vi "NFC Mngr.vi"(7 "Mngr Action":T1, 8 "error in (no error)":errorcluster, 10 "Python Version":string, 11 "Reader SN":string="21121521200223") -> (0 "error out":errorcluster, 3 "Cartridge SN":string, 4 "Connected":bool)   [LabVIEW 2018]
uses:
  NFC Mngr.ctl
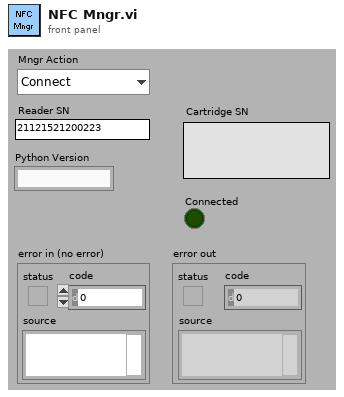
[diagram p1: front panel]
types:
  T1 = typedef "NFC Mngr.ctl" = enum16{"Connect", "Read SN", "Close"}
  T2 = enum16{"Init", "Reset", "Read", "Update", "Close"}
  T3 = cluster{"negative limit switch":bool, "positive limit switch":bool, "home switch":bool, "position marker":bool, "device enable":bool, "quick stop":bool, "general purpose J":bool, "general purpose I":bool, "general purpose H":bool, "general purpose G":bool, "general purpose F":bool, "general purpose E":bool, "general purpose D":bool, "general purpose C":bool, "general purpose B":bool, "general purpose A":bool}
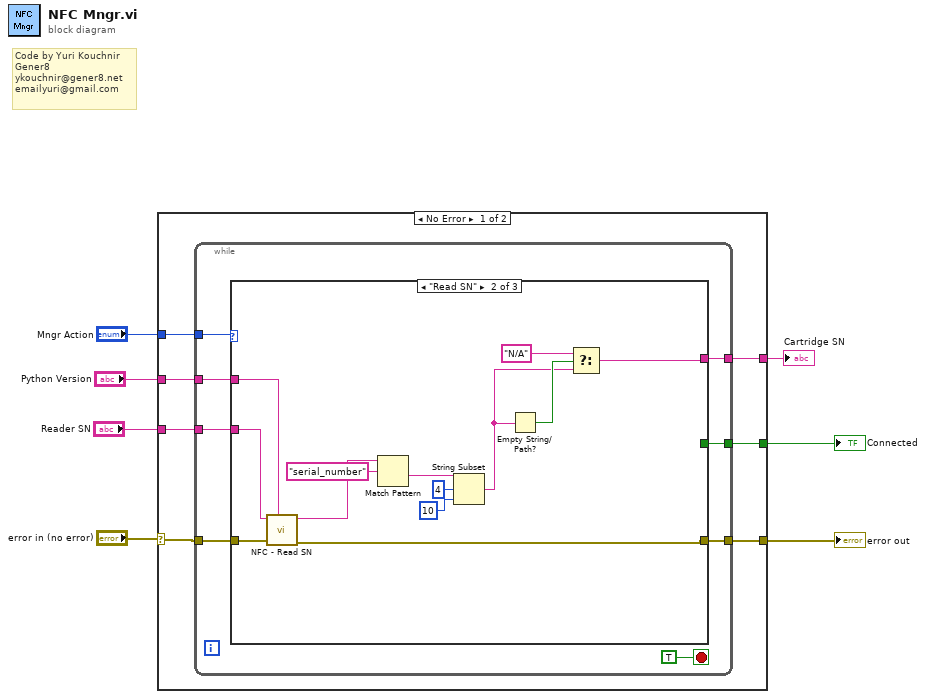
[diagram p0: block diagram]
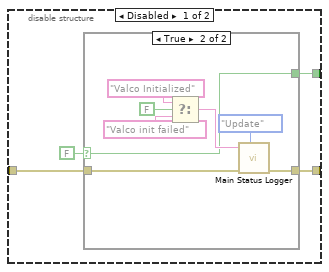
[diagram p3: hidden frame]
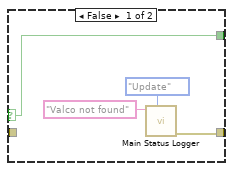
[diagram p4: hidden frame]
diagram:
  # "Code by Yuri Kouchnir\nGener8\nykouchnir@gener8.net\nemailyuri@gmail.com"
  n1 = case shown="No Error" "error in (no error)" {
    selector: "error in (no error)" -> [w14 w57]
    tunnel: [w13 w57] -> w6
    tunnel: "Mngr Action" -> [w12 _]
    tunnel: [w11 _] -> w4
    tunnel: "Reader SN" -> [w10 _]
    tunnel: [w9 _] -> w2
    tunnel: "Python Version" -> [w8 _]
    frame No Error {
      n2 = while {
        tunnel: w14 -> [w20]
        tunnel: [w19] -> w13
        tunnel: w12 -> [w21]
        tunnel: [w18] -> w11
        tunnel: w10 -> [w17]
        tunnel: [w16] -> w9
        tunnel: w8 -> [w15]
        stop <- TRUE stop-if-true
        n3 = case shown="\"Read SN\"" w21 {
          tunnel: w20 -> [w23 w55 w56]
          tunnel: [w25 w54 w56] -> w19
          tunnel: [w24 _ _] -> w18
          tunnel: w17 -> [_ w53 _]
          tunnel: [_ w44 _] -> w16
          tunnel: w15 -> [_ w43 _]
          frame "Connect" {
            n4 = disable-structure shown="Enabled" {
              disable-tunnel: [w29 w42] -> w25
              disable-tunnel: [w28 _] -> w24
              disable-tunnel: w23 -> [w27 w42]
              frame Disabled {
                n5 = case shown="True" FALSE {
                  selector: FALSE -> [w33 w36]
                  tunnel: [w31 w37] -> w29
                  tunnel: [w33 w36] -> w28
                  tunnel: w27 -> [_ w34]
                  frame False {
                    n6 = call "Main Status Logger.vi"("Action"=T2."Update", "Input String"="Valco not found") -> ("error out"=w31:errorcluster)  [unwired: 8 in, 1 out]
                  }
                  frame True {
                    n7 = Select(t="Valco Initialized" ("ID Response"), s=FALSE, f="Valco init failed" ("ID Response")) -> (s? t:f=w38:string)
                    n8 = call "Main Status Logger.vi"("Action"=T2."Update", "error in"=w34, "Input String"=w38) -> ("error out"=w37:errorcluster)  [unwired: 7 in, 1 out]
                  }
                }
              }
              frame Enabled {
              }
            }
          }
          frame "Read SN" {
            n9 = call "NFC - Read SN.vi"("Python Version"=w43, "error in (no error)"=w55, "Reader SN"=w53) -> ("error out"=w54:errorcluster, "Cartridge SN"=w48:string)  [unwired: 7 in]
            n10 = Match Pattern(string=w48, regular expression="serial_number") -> (after substring=w51:string)  [unwired: 1 in, 3 out]
            n11 = String Subset(string=w51, offset (0)=4, length (rest)=10 ("length (rest)")) -> (substring=w45:string)
            n12 = Empty String/Path?(string/path=w45) -> (empty?=w47:bool)
            n13 = Select(t="N/A" ("regular expression"), s=w47, f=w45) -> (s? t:f=w44:string)
          }
          frame "Close" {
          }
        }
      }
    }
    frame Error {
      (unwired) T3 {"negative limit switch"=FALSE, "positive limit switch"=FALSE, "home switch"=FALSE, "position marker"=FALSE, "device enable"=FALSE, "quick stop"=FALSE, "general purpose J"=FALSE, "general purpose I"=FALSE, "general purpose H"=FALSE, "general purpose G"=FALSE, "general purpose F"=FALSE, "general purpose E"=FALSE, "general purpose D"=FALSE, "general purpose C"=FALSE, "general purpose B"=FALSE, "general purpose A"=FALSE} ("digital inputs")
    }
  }
  "error out" <- w6
  "Connected" <- w4
  "Cartridge SN" <- w2
